vi "TemplateImageToTopEdge (SubVI).vi"(6 "Line Fit Options":T2={"Number of Lines"=1, "Type"=enum."First Edge Rake", "Min. Score"=10.0, "Max. Score"=1000.0, "Orientation"=0.0, "Angle Range"=45.0, "Angle Tolerance"=1.0, "Step Size"=7, "Min. SNR (db)"=0.0, "Min. Points (%)"=25.0, "Hough Iterations"=5} {"Min. Points (%)" min=0.0 max=100.0; "Min. SNR (db)" min=0.0; "Max. Score" min=0.0 max=1024.0; "Min. Score" min=0.0 max=1024.0 step=1.0}, 7 "Pattern Match Settings":T11={"Algorithm"=2, "Number of Matches Requested"=1, "Minimum Match Score"=700.0, "SubPixel Accuracy"=TRUE, "Rotation Angle Ranges"=[{"Start"=-90.0, "End"=90.0}], "Show Search Area"=FALSE, "Show Result"=TRUE} {"Rotation Angle Ranges"."End" format="%.1f"; "Rotation Angle Ranges"."Start" format="%.1f"; "Minimum Match Score" min=0 max=1000 format="%.2f"; "Number of Matches Requested" min=1; "Algorithm" items=["All", "Low Discrepancy Sampling", "Grayscale Value Pyramid", "Gradients Pyramid"]}, 8 "error in (no error)":errorcluster, 9 "Calibrated Image":T8, 10 "Search Rect":T10={"Left"=0, "Top"=0, "Right"=2147483647, "Bottom"=2147483647, "Rotation"=0.0} {"Rotation" format="%.2f"; "Left" scale=0.0..1024.0; "Right" scale=0.0..1024.0}, 11 "GenClassTagFlatRef in":refnum<vi>) -> (0 "error out":errorcluster, 1 "Straight Edges":T1(array[cluster]) {"Point2 (Real-World)"."Y" format="%.2f"; "Point2 (Real-World)"."X" format="%.2f"; "Point1 (Real-World)"."Y" format="%.2f"; "Point1 (Real-World)"."X" format="%.2f"; "Point2 (Pixels)"."Y" format="%.2f"; "Point2 (Pixels)"."X" format="%.2f"; "Point1 (Pixels)"."Y" format="%.2f"; "Point1 (Pixels)"."X" format="%.2f"}, 2 "ROI Descriptor after matches":T9, 3 "Refnum out":T8)   [LabVIEW 2016]
uses:
  <vilib>/vision/Image Controls.llb/IMAQ Image.ctl
  <vilib>/vision/Measure.llb/Edge Options.ctl
  <vilib>/vision/Measure.llb/Edge Polarity.ctl
  <vilib>/vision/Measure.llb/Straight Edge Options.ctl
  <vilib>/vision/Measure.llb/Straight Edge Process.ctl
  <vilib>/vision/NI_Vision_Development_Module.lvlib
  <resource>/objmgr/IMAQImage.rc
panel:
  in  "Options: Top Edge Search":T6={"Search Direction"=2, "Edge Options"={"Edge Polarity"=0, "Kernel Size"=9, "Width"=3, "Minimum Edge Strength"=17.0, "Interpolation Type"=enum."Bilinear Fixed", "Data Processing Method"=enum."Average"}, "Show Search Area"=TRUE, "Show Search Lines"=TRUE, "Show Edges Found"=TRUE, "Show Result"=TRUE, "Search Area Color"=65280, "Search Lines Color"=255, "Edge Locations Color"=16776960, "Result Color"=16711680, "Overlay Group Name"=""} {"Search Direction" items=["Left to Right", "Right to Left", "Top to Bottom", "Bottom to Top"]; "Edge Options"."Edge Polarity" items=["All Edges", "Rising Edges", "Falling Edges"]; "Edge Options"."Minimum Edge Strength" format="%.2f"; "Edge Options"."Width" step=2; "Edge Options"."Kernel Size" step=2}
  in  "ROI Descriptor before matches":T7={"Global Rectangle"=[675, 567, 1751, 1642], "Contours"=[{"ID"=enum."External", "Type"=12, "Coordinates"=[1212, 1104, 85, 537, 0, 0]}]} {"Contours"."Type" items=["No Selection", "Point", "Line", "Rectangle", "Oval", "Polygon", "Freehand Region", "Annulus", "Unused2", "Unused3", "Broken Line", "Freehand Line", "Rotated Rectangle"]}
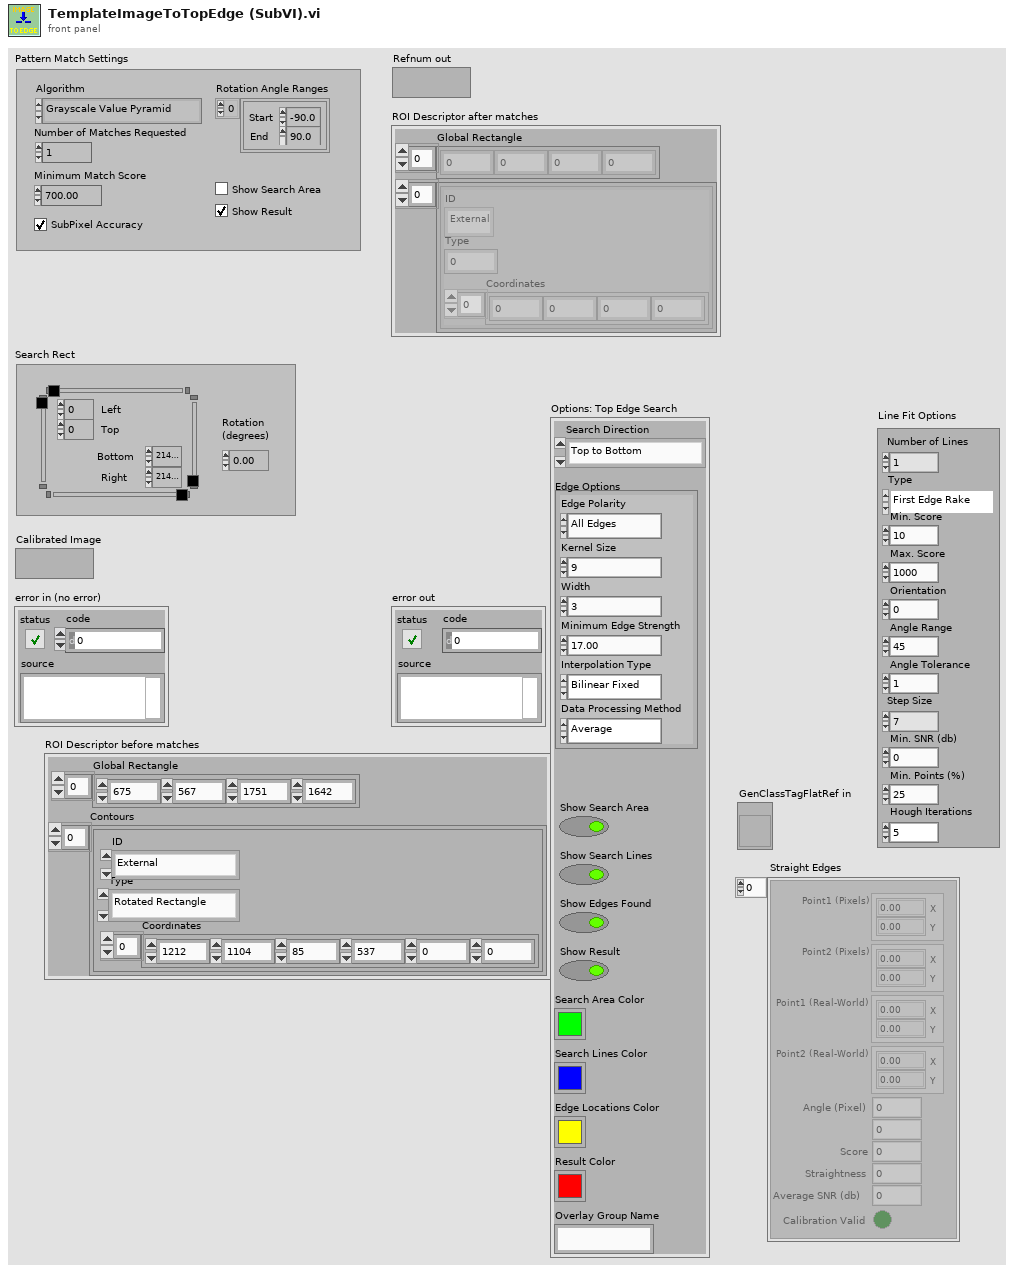
[diagram p1: front panel]
types:
  T1 = cluster{"Point1 (Pixels)":cluster{"X":sgl, "Y":sgl}, "Point2 (Pixels)":cluster{"X":sgl, "Y":sgl}, "Point1 (Real-World)":cluster{"X":sgl, "Y":sgl}, "Point2 (Real-World)":cluster{"X":sgl, "Y":sgl}, "Angle (Pixel)":dbl, "Angle (Real-World)":dbl, "Score":dbl, "Straightness":dbl, "Average SNR (db)":dbl, "Calibration Valid":bool}[]
  T2 = typedef "Straight Edge Options.ctl" = cluster{"Number of Lines":i32, "Type":T3, "Min. Score":dbl, "Max. Score":dbl, "Orientation":dbl, "Angle Range":dbl, "Angle Tolerance":dbl, "Step Size":u32, "Min. SNR (db)":dbl, "Min. Points (%)":dbl, "Hough Iterations":i32}
  T3 = typedef "Straight Edge Process.ctl" = enum32{"First Edge Rake", "Best Edge Rake", "Hough Edge Rake", "First Edge Projection", "Best Edge Projection"}
  T4 = typedef "Edge Options.ctl" = cluster{"Edge Polarity":T5, "Kernel Size":u32, "Width":u32, "Minimum Edge Strength":sgl, "Interpolation Type":enum32{"Zero Order", "Bilinear", "Quadratic", "Cubic", "Bilinear Fixed"}, "Data Processing Method":enum32{"Average", "Median"}}
  T5 = typedef "Edge Polarity.ctl" = u32
  T6 = cluster{"Search Direction":u32, "Edge Options":T4, "Show Search Area":bool, "Show Search Lines":bool, "Show Edges Found":bool, "Show Result":bool, "Search Area Color":u32, "Search Lines Color":u32, "Edge Locations Color":u32, "Result Color":u32, "Overlay Group Name":string}
  T7 = cluster{"Global Rectangle":i32[], "Contours":cluster{"ID":enum32{"External", "Internal"}, "Type":u32, "Coordinates":i32[]}[]}
  T8 = typedef "IMAQ Image.ctl" = refnum<image>
  T9 = cluster{"Global Rectangle":i32[], cluster{"ID":enum32{"External", "Internal"}, "Type":u32, "Coordinates":i32[]}[]}
  T10 = typedef "IMAQ Rectangle" = cluster{"Left":i32, "Top":i32, "Right":i32, "Bottom":i32, "Rotation":dbl}
  T11 = cluster{"Algorithm":i32, "Number of Matches Requested":i32, "Minimum Match Score":sgl, "SubPixel Accuracy":bool, "Rotation Angle Ranges":cluster{"Start":sgl, "End":sgl}[], "Show Search Area":bool, "Show Result":bool}
  T12 = cluster{"Left":i32, "Top":i32, "Right":i32, i32, "Rotation":dbl}
  T13 = cluster{"Position":cluster{"x":sgl, "y":sgl}, "Angle":sgl, "Scale":sgl, "Score":sgl, "Bounding Box":cluster{"x":sgl, "y":sgl}[]}[]
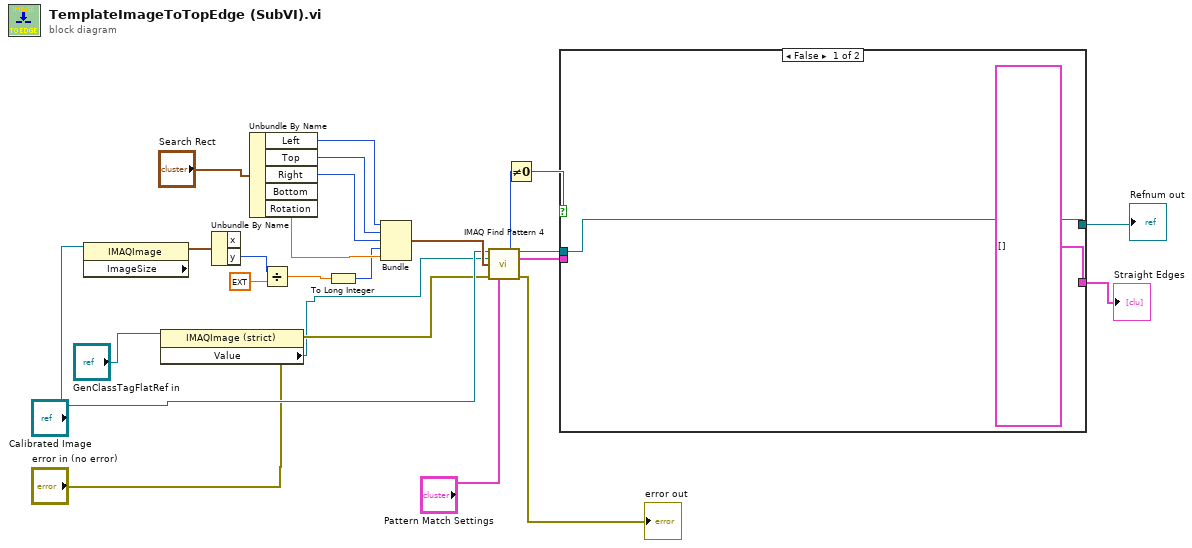
[diagram p0: block diagram]
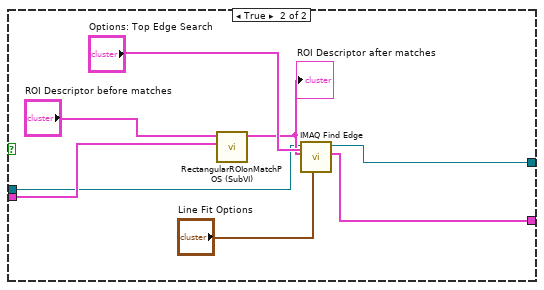
[diagram p2: hidden frame]
diagram:
  n1 = property class="IMAQImage"(reference="Calibrated Image") -> ("ImageSize"=w21:cluster{"x":i32, "y":i32})  [unwired: 1 in, 2 out]
  n2 = property class="IMAQImage (strict)"(reference="GenClassTagFlatRef in") -> ("Value"=w11:T8)  [unwired: 1 in, 2 out]
  n3 = Unbundle By Name(w21) -> ("y"=w9:i32)  [unwired: 1 out]
  n4 = Unbundle By Name("Search Rect") -> ("Left"=w19:i32, "Top"=w20:i32, "Right"=w13:i32, "Rotation"=w12:dbl)  [unwired: 1 out]
  n5 = Divide(x=w9, y=ext 2.5) -> (x/y=w7:ext)
  n6 = To Long Integer(number=w7) -> (32bit integer=w6:i32)
  n7 = Bundle("Left"=w19, "Top"=w20, "Right"=w13, w6, "Rotation"=w12) -> (w23:T12)  [unwired: 1 in]
  n8 = call "IMAQ Find Pattern 4"("Image"="Calibrated Image", "Template"=w11, "Search Rect"=w23, "error in"="error in (no error)", "Settings"="Pattern Match Settings") -> ("Number of Matches"=w3:i32, "Image Out"=w5:T8, "Matches (pixel)"=w17:T13, "error out"=→"error out":errorcluster)  [unwired: 4 in, 3 out]
  n9 = Not Equal To 0?(x=w3) -> (x != 0?=w4:bool)
  n10 = case shown="False" w4 {
    tunnel: w17 -> [_ w33]
    tunnel: w5 -> [w24 w28]
    tunnel: [w24 w27] -> w2
    tunnel: [T1 [] ("Straight Edges") w26] -> w1
    frame False {
    }
    frame True {
      n11 = call "RectangularROIonMatchPOS (SubVI).vi"("Matches (pixel)"=w33, "ROI Descriptor before matches"="ROI Descriptor before matches") -> ("ROI Descriptor after matches"=w29:T9)  [unwired: 8 in, 1 out]
      "ROI Descriptor after matches" <- w29
      n12 = call "IMAQ Find Edge"("Line Fit Options"="Line Fit Options", "Options"="Options: Top Edge Search", "ROI Descriptor"=w29, "Image"=w28) -> ("Straight Edges"=w26:T1, "Image Out"=w27:T8)  [unwired: 4 in, 2 out]
    }
  }
  "Refnum out" <- w2
  "Straight Edges" <- w1
